vi "CRYStep Pic Save SetupView .vi"(8 "nIDV":i32, 9 "sStepName":string) -> ()   [LabVIEW 2013]
uses:
  CRYProject Editor Global.vi
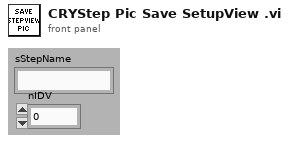
[diagram p1: front panel]
types:
  T1 = typedef "CRYTS.ctl" = cluster{"No.TS":u16, "TS File Path":path, "TS Name":string, "EditStepName":string, "Steps":T2[], "New State":bool, "Change State":bool, "Flattened CurveLib Data":string, "Document Data":string, "EditStepNo":u16, "Operator Start File":string, "Sequence Type":string, "Sequence Language":string}
  T2 = typedef "CRYStep.ctl" = cluster{"No.VI":i32, "Category":string, "StepName":string, "Seq setup flattened":string, "Comment":string, "Steps config.":bool[], "Jump config":i32[], "Start":dbl, "Increment":dbl, "Name":string, "Unit":string, "Y data":u16, "Y prefix":string, "Y dB ref":dbl, "Y unit":string, "Repeat State Array":cluster{"Start":dbl, "Increment":dbl, "Count":i32, "Num":i32}[]}
  T3 = cluster{"nID":i32, "sName":string, "sType":string, "sProperty":string, "sTemplet":string, "sDocking":string, "pVIRef":refnum<vi>, "pSPRef":refnum<vi>, "pRefTemplet":refnum<vi>, "pRefSplitter":refnum<vi>[], "nPosSplitter":i32[], "pRefSP":refnum<vi>[], "nSPID":i32[], "sSPDock":string[], "nIDFrame":i32[], "nIDPanel":i32[], "nActiveFrame":i32, "nCountFrame":i32, "cFrame":cluster{"nID":i32, "sName":string, "sType":string, "sTitle":string, "sIcon":string, "pVIRef":refnum<vi>, "pSPRef":refnum<vi>, "cWiin":cluster{"sName":string, "sType":string, "pVIRef":refnum<vi>, "sData":string}, "cTab":cluster{"sTitle":string, "sIcon":string, "pSpliter":refnum<vi>, "nAvtivePage":i32, "nIDPage":i32[], "nIDFrame":i32[]}, "sData":string}[], "sData":string, "sSplitterName":string[]}
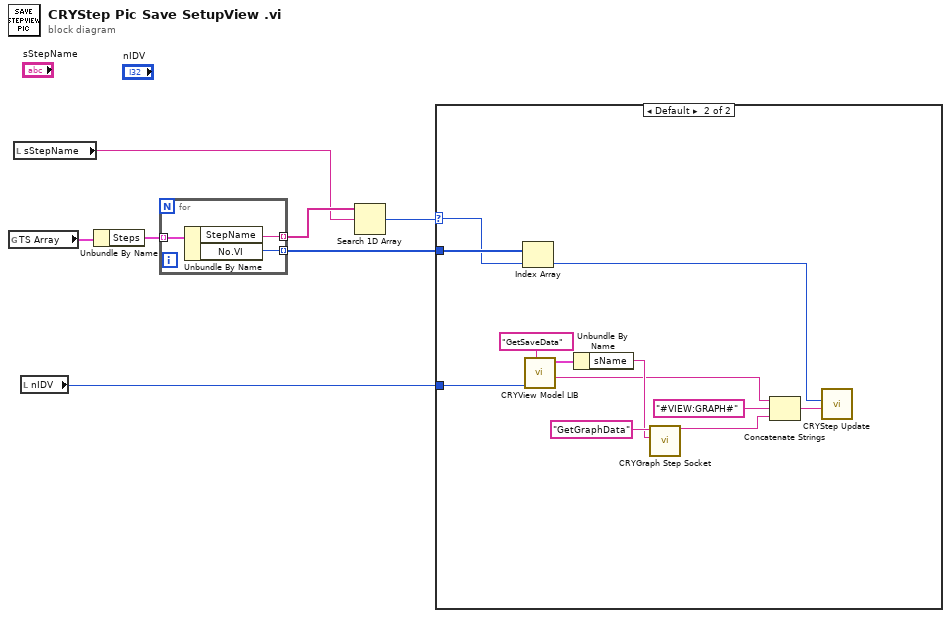
[diagram p0: block diagram]
diagram:
  n1 = global read "CRYProject Editor Global.vi" "TS Array"() -> (w5:T1)
  n2 = local read "sStepName"() -> (w3:string)
  n3 = local read "nIDV"() -> (w7:i32)
  n4 = Unbundle By Name(w5) -> ("Steps"=w6:T2[])
  n5 = for {
    tunnel: w6 -> [w10] mode=indexing
    tunnel: [w9] -> w4 mode=indexing
    tunnel: [w8] -> w1 mode=indexing
    n6 = Unbundle By Name(w10) -> ("StepName"=w9:string, "No.VI"=w8:i32)
  }
  n7 = Search 1D Array(1D array=w4, element=w3) -> (index of element=w2:i32)  [unwired: 1 in]
  n8 = case shown="Default" w2 {
    selector: w2 -> [_ w12]
    tunnel: w7 -> [_ w16]
    tunnel: w1 -> [_ w13]
    frame -1 {
    }
    frame Default {
      n9 = Index Array(array=w13, index=w12) -> (element=w11:i32)
      n10 = call "CRYView Model LIB.vi"("sAction"="GetSaveData", "nData"=w16) -> ("sData_Out"=w15:string, "cView_Out"=w20:T3)  [unwired: 7 in, 1 out]
      n11 = Unbundle By Name(w20) -> ("sName"=w19:string)
      n12 = call "CRYGraph Step Socket.vi"("Queue Name"=w19, "sAction"="GetGraphData") -> ("sDataOut"=w14:string)  [unwired: 9 in]
      n13 = Concatenate Strings(w15, "#VIEW:GRAPH#" ("regular expression"), w14) -> (w17:string)
      n14 = call "CRYStep Update.vi"("Seq-step setup"=w17, "Proper VI No"=w11) -> ()  [unwired: 5 in, 5 out]
    }
  }
